vi "PutArrayLen.vi"(8 "error in (no error)":errorcluster, 10 "len":i32, 11 "MsgPackSerializer in":refnum<class "MsgPackSerializer.lvclass">) -> (0 "error out":errorcluster, 3 "MsgPackSerializer out":refnum<class "MsgPackSerializer.lvclass">)   [LabVIEW 2015, in "MsgPackSerializer.lvclass"]
uses:
  MsgPackSerializer.lvclass
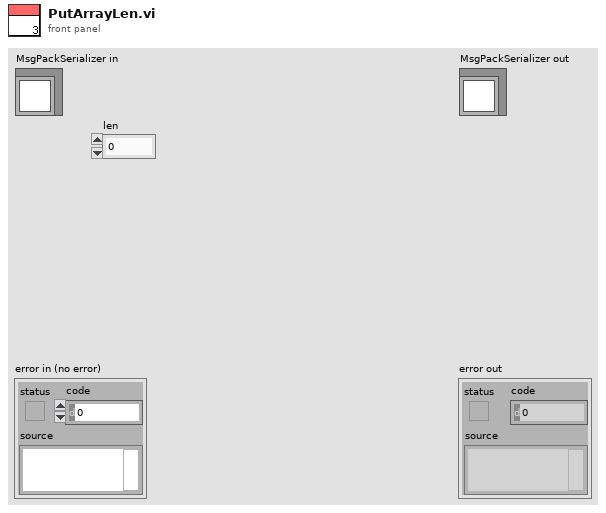
[diagram p1: front panel]
types:
  T1 = enum16{"big-endian, network order", "native, host order", "little-endian"}
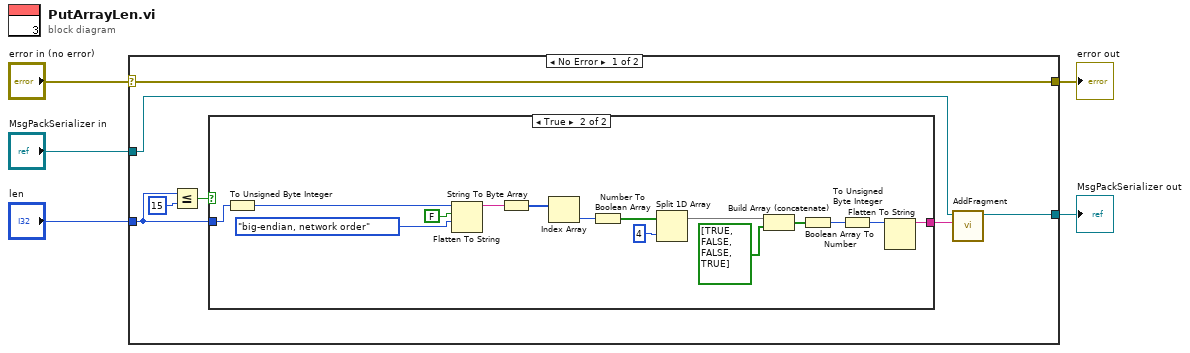
[diagram p0: block diagram]
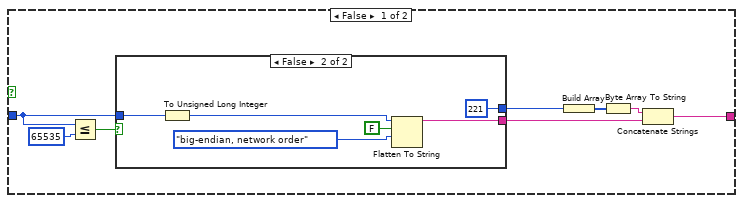
[diagram p2: hidden frame]
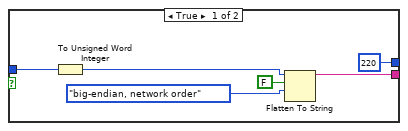
[diagram p3: hidden frame]
diagram:
  n1 = case shown="No Error" "error in (no error)" {
    selector: "error in (no error)" -> [w12 w49]
    tunnel: [w12 w49] -> w4
    tunnel: [w7 w48] -> w2
    tunnel: "MsgPackSerializer in" -> [w8 w48]
    tunnel: "len" -> [w9 _]
    frame No Error {
      n2 = Less Or Equal?(x=w9, y=15) -> (x <= y?=w11:bool)
      n3 = case shown="True" w11 {
        tunnel: w9 -> [w18 w43]
        tunnel: [w13 w38] -> w6
        frame False {
          n4 = Less Or Equal?(x=w18, y=65535) -> (x <= y?=w19:bool)
          n5 = case shown="False" w19 {
            tunnel: w18 -> [w26 w32]
            tunnel: [u8 220 ("Number") u8 221 ("Number")] -> w15
            tunnel: [w21 w27] -> w14
            frame True {
              n6 = To Unsigned Word Integer(number=w26) -> (unsigned 16bit integer=w23:u16)
              n7 = Flatten To String(anything=w23, prepend array or string size? (T)=FALSE, byte order (0:big-endian, network order)=T1."big-endian, network order") -> (data string=w21:string)  [unwired: 1 in, 2 out]
            }
            frame False {
              n8 = To Unsigned Long Integer(number=w32) -> (unsigned 32bit integer=w29:u32)
              n9 = Flatten To String(anything=w29, prepend array or string size? (T)=FALSE, byte order (0:big-endian, network order)=T1."big-endian, network order") -> (data string=w27:string)  [unwired: 1 in, 2 out]
            }
          }
          n10 = Build Array(w15) -> (w17:u8[])
          n11 = Byte Array To String(unsigned byte array=w17) -> (string=w16:string)
          n12 = Concatenate Strings(w16, w14) -> (w13:string)
        }
        frame True {
          n13 = To Unsigned Byte Integer(number=w43) -> (unsigned 8bit integer=w42:u8)
          n14 = Flatten To String(anything=w42, prepend array or string size? (T)=FALSE, byte order (0:big-endian, network order)=T1."big-endian, network order") -> (data string=w45:string)  [unwired: 1 in, 2 out]
          n15 = String To Byte Array(string=w45) -> (unsigned byte array=w44:u8[])
          n16 = Index Array(array=w44) -> (element=w41:u8)  [unwired: 1 in]
          n17 = Number To Boolean Array(number=w41) -> (Boolean array=w39:bool[])
          n18 = Split 1D Array(array=w39, index=4) -> (first subarray=w37:bool[])  [unwired: 1 out]
          n19 = Build Array (concatenate)(w37, bool[] [TRUE, FALSE, FALSE, TRUE] ("Boolean array")) -> (w35:bool[])
          n20 = Boolean Array To Number(Boolean array=w35) -> (number=w34:u32)
          n21 = To Unsigned Byte Integer(number=w34) -> (unsigned 8bit integer=w33:u8)
          n22 = Flatten To String(anything=w33) -> (data string=w38:string)  [unwired: 3 in, 2 out]
        }
      }
      n23 = call "AddFragment.vi"("Fragment"=w6, "MsgPackSerializer in"=w8) -> ("MsgPackSerializer out"=w7:refnum<class "MsgPackSerializer.lvclass">)  [unwired: 8 in, 1 out]
    }
    frame Error {
    }
  }
  "error out" <- w4
  "MsgPackSerializer out" <- w2
